vi "Initialize SharedRsc Attribute.vi"() -> (3 "Attribute.SharedResource":refnum<class "Attribute.SharedResource.lvclass">)   [LabVIEW 2019, in "Attribute.SharedResource.lvclass"]
doc: "JKI State Machine Objects (SMO) 1.3.0.56\nJKI - JKI\nCopyright (c) 2017, JKI"
uses:
  Attribute.SharedResource.lvclass
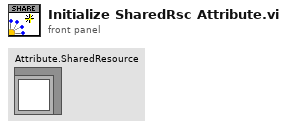
[diagram p1: front panel]
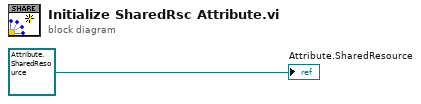
[diagram p0: block diagram]
diagram:
  "Attribute.SharedResource" <- refnum<class "Attribute.SharedResource.lvclass"> refnum ("Attribute.Owner in")
